vi "Insert into Subpanel.vi"(8 "error in (no error)":errorcluster, 10 "SubPanel":refnum<vi>, 11 "Malleable VI Type in":refnum<class "Malleable VI Type.lvclass">) -> (0 "error out":errorcluster, 3 "Malleable VI Type out":refnum<class "Malleable VI Type.lvclass">)   [LabVIEW 2020, in "Peek Window.lvlib" / "Malleable VI Type.lvclass"]
uses:
  Malleable VI Type.lvclass
  Malleable VI Type.lvclass/Malleable VI Type.ctl
  Standard VI Type/Standard VI Type.lvclass/Standard VI Type.ctl
  Standard VI Type/Read VI Refnum.vi
  Implementation VI Type/Implementation VI Type.lvclass
  D:/Code/VI-Peek/source/Peek Window/VI Types/Standard VI Type/Standard VI Type.lvclass
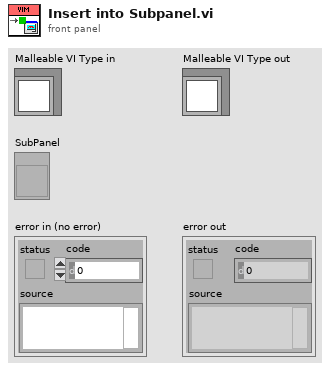
[diagram p1: front panel]
types:
  T1 = enum8{"Enabled", "Disabled", "Disabled and Grayed Out"}
  T2 = typedef "Peek Window.lvlib/Malleable VI Type.lvclass/Selected Implementation Enum.ctl" = enum16{"Actual", "Instance"}
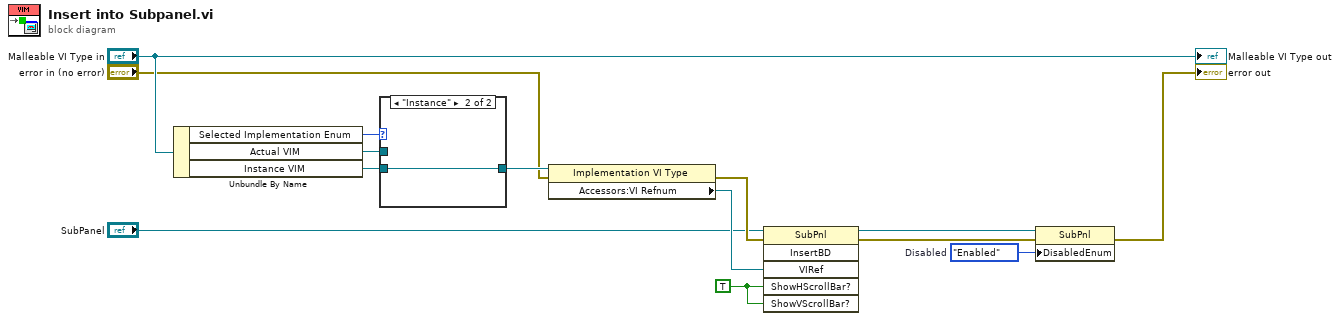
[diagram p0: block diagram]
diagram:
  w4 = T1."Enabled"  # Disabled
  w10 = TRUE ("ShowHScrollBar")
  n1 = Unbundle By Name("Malleable VI Type in") -> ("Selected Implementation Enum"=w13:T2, "Actual VIM"=w12:refnum<class "Implementation VI Type.lvclass">, "Instance VIM"=w11:refnum<class "Implementation VI Type.lvclass">)
  n2 = case shown="\"Instance\"" w13 {
    tunnel: w12 -> [w15 _]
    tunnel: w11 -> [_ w16]
    tunnel: [w15 w16] -> w7
    frame "Actual" {
    }
    frame "Instance" {
    }
  }
  n3 = property class="Implementation VI Type"(reference=w7, error in="error in (no error)") -> (error out=w8:errorcluster, "Accessors:VI Refnum"=w9:refnum<vi>)  [unwired: 1 out]
  n4 = invoke on="Invoke Node" class="SubPnl" method="InsertBD"(reference="SubPanel", error in=w8, "VIRef"=w9, "ShowHScrollBar?"=w10, "ShowVScrollBar?"=w10) -> (reference out=w3:refnum<vi>, error out=w2:errorcluster)  [unwired: 1 in, 4 out]
  n5 = property class="SubPnl"(reference=w3, error in=w2, "DisabledEnum"=w4) -> (error out=→"error out":errorcluster)  [unwired: 1 out]
  "Malleable VI Type out" <- "Malleable VI Type in"
